vi "Player Info.vi"(11 "Awesome! in":refnum<class "Awesome!.lvclass">) -> (0 "Defeat Speech":string, 1 "Victory Speech":string, 2 "Name":string, 3 "Awesome! out":refnum<class "Awesome!.lvclass">)   [LabVIEW 2016, in "Awesome!.lvclass"]
uses:
  Awesome!.lvclass
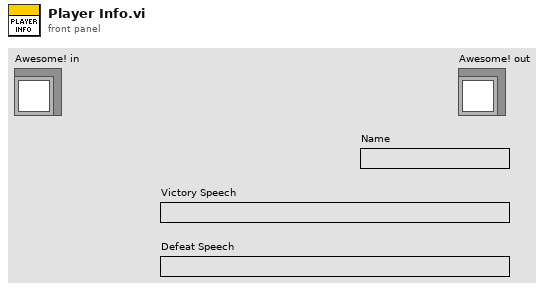
[diagram p1: front panel]
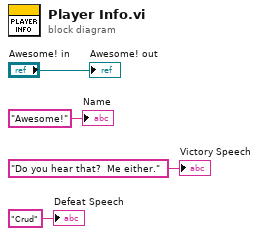
[diagram p0: block diagram]
diagram:
  "Awesome! out" <- "Awesome! in"
  "Name" <- "Awesome!" ("Name")
  "Victory Speech" <- "Do you hear that?  Me either." ("Victory Speech")
  "Defeat Speech" <- "Crud" ("Defeat Speech")
